vi "Template - DMM Acquire Triggered Multiple.vi"() -> ()   [LabVIEW 2015]
doc: "This example shows how to configure a measurement, set up triggering, trigger a measurement, and retrieve a measurement. It shows how to use the low-level Data VIs to retrieve data from the DMM."
uses:
  <instrlib>/_Template - DMM/Template - DMM.lvlib
panel:
  in  "Function (0: DC Volts)":u16(ring) items=["DC Volts", "AC Volts", "DC Current", "AC Current", "2-Wire Resistance", "4-Wire Resistance"]
  in  "Serial Configuration":T1={"Baud Rate"=9600, "Parity"=0, "Data Bits"=7, "Stop Bits"=10, "Flow Control"=0} {"Flow Control" items=["None", "XON/XOFF", "RTS/CTS", "XON/XOFF & RTS/CTS", "DTR/DSR", "XON/XOFF & DTR/DSR"]; "Stop Bits" items=["1.0"=10, "1.5"=15, "2.0"=20]; "Data Bits" items=["7"=7, "8"=8]; "Parity" items=["None", "Odd", "Even", "Mark", "Space"]; "Baud Rate" items=["300"=300, "600"=600, "1200"=1200, "2400"=2400, "4800"=4800, "9600"=9600, "19200"=19200]}
  in  "Sample Count (10)":i32=10 format="%#.6g"
  in  "Timeout (10000 ms)":i32=10000 format="%#.6g"
  in  "Trigger Count (5)":i32=5 format="%#.6g"
  out "Waveform Chart":dbl[][](graph)
  in  "VISA resource name":refnum<visa-resource-name>
  # "(c) 2014 <Enter Company Name Here>.  ALL RIGHTS RESERVED."
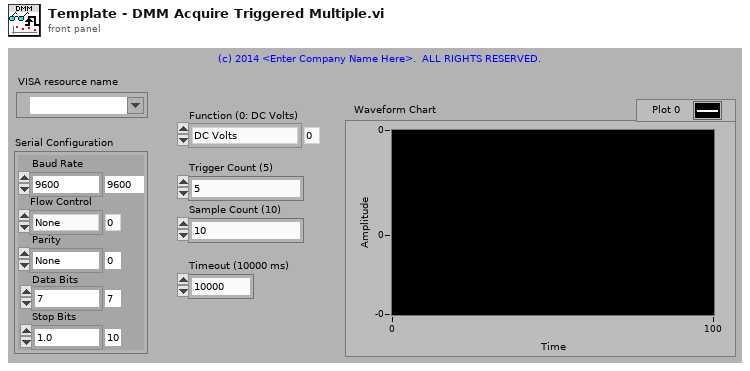
[diagram p1: front panel]
types:
  T1 = cluster{"Baud Rate":u32, "Parity":u16, "Data Bits":u16, "Stop Bits":u16, "Flow Control":u16}
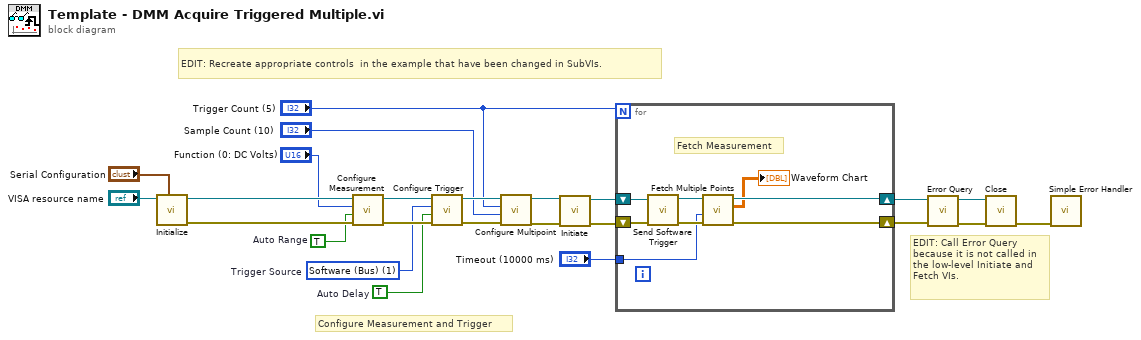
[diagram p0: block diagram]
diagram:
  w11 = u16 1 items=["Immediate", "Software (Bus)", "External"]  # Trigger Source
  w12 = TRUE  # Auto Range
  w13 = TRUE  # Auto Delay
  # "EDIT: Call Error Query because it is not called in the low-level Initiate and Fetch VIs."
  # "EDIT: Recreate appropriate controls  in the example that have been changed in SubVIs."
  # "Configure Measurement and Trigger"
  n1 = call <instrlib>:"Initialize.vi"("Serial Configuration"="Serial Configuration", "VISA resource name"="VISA resource name") -> ("error out"=w22:errorcluster, "VISA resource name out"=w23:refnum<visa-resource-name>)  [unwired: 8 in]
  n2 = call <instrlib>:"Configure Measurement.vi"("error in (no error)"=w22, "Auto Range (T:Enable)"=w12, "Function (0: DC Volts)"="Function (0: DC Volts)", "VISA resource name"=w23) -> ("error out"=w20:errorcluster, "VISA resource name out"=w21:refnum<visa-resource-name>)  [unwired: 6 in]
  n3 = call <instrlib>:"Configure Trigger.vi"("error in (no error)"=w20, "Auto Delay (T:Enable)"=w13, "Trigger Source (0: Immediate)"=w11, "VISA resource name"=w21) -> ("error out"=w18:errorcluster, "VISA resource name out"=w19:refnum<visa-resource-name>)  [unwired: 6 in]
  n4 = call <instrlib>:"Configure Multipoint.vi"("error in (no error)"=w18, "Sample Count (1)"="Sample Count (10)", "Trigger Count (1)"="Trigger Count (5)", "VISA resource name"=w19) -> ("error out"=w9:errorcluster, "VISA resource name out"=w10:refnum<visa-resource-name>)  [unwired: 6 in]
  n5 = call <instrlib>:"Initiate.vi"("error in (no error)"=w9, "VISA resource name"=w10) -> ("error out"=w8:errorcluster, "VISA resource name out"=w7:refnum<visa-resource-name>)  [unwired: 8 in]
  n6 = for {
    N: "Trigger Count (5)" -> [_]
    shift-right: [w31] -> w3
    shift-left: w8 -> [w27]
    tunnel: "Timeout (10000 ms)" -> [w26]
    shift-right: [w32] -> w5
    shift-left: w7 -> [w28]
    # "Fetch Measurement"
    n7 = call <instrlib>:"Send Software Trigger.vi"("error in (no error)"=w27, "VISA resource name"=w28) -> ("error out"=w29:errorcluster, "VISA resource name out"=w30:refnum<visa-resource-name>)  [unwired: 8 in]
    n8 = call <instrlib>:"Fetch Multiple Points.vi"("error in (no error)"=w29, "Timeout (10000 ms)"=w26, "VISA resource name"=w30) -> ("error out"=w31:errorcluster, "Measurements"=→"Waveform Chart":dbl[][], "VISA resource name out"=w32:refnum<visa-resource-name>)  [unwired: 6 in]
  }
  n9 = call <instrlib>:"Error Query.vi"("error in (no error)"=w3, "VISA resource name"=w5) -> ("error out"=w2:errorcluster, "VISA resource name out"=w4:refnum<visa-resource-name>)  [unwired: 6 in, 2 out]
  n10 = call <instrlib>:"Close.vi"("error in (no error)"=w2, "VISA resource name"=w4) -> ("error out"=w16:errorcluster)  [unwired: 9 in]
  n11 = call <vilib>:"Simple Error Handler.vi"("error in (no error)"=w16) -> ()  [unwired: 4 in, 5 out]
